vi "Read DL_param.vi"(8 "error in (no error)":errorcluster, 11 "Control-Client in":refnum<class "Control-Client.lvclass">) -> (0 "error out":errorcluster, 2 "DL_param":T1={"min I, mm"=-900.0, "max I, mm"=100.0, "Real Optical 0, ps"=480.0, "min II, mm"=-70.0, "max II, mm "=50.0}, 3 "Control-Client out":refnum<class "Control-Client.lvclass">)   [LabVIEW 2015, in "Control-Client.lvclass"]
uses:
  Control-Client.lvclass
  Control-Client.lvclass/Control-Client.ctl
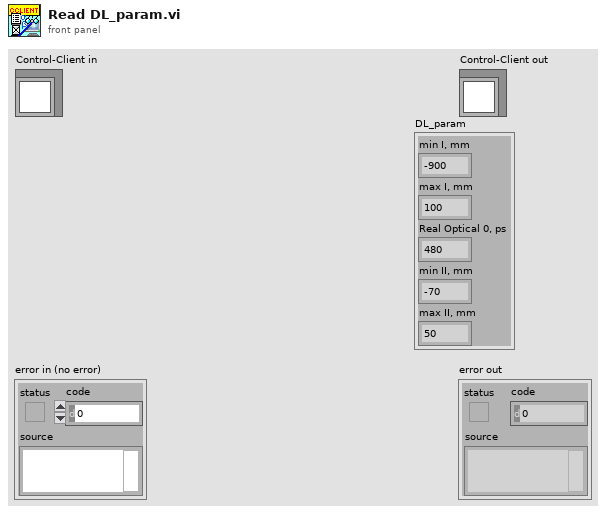
[diagram p1: front panel]
types:
  T1 = cluster{"min I, mm":dbl, "max I, mm":dbl, "Real Optical 0, ps":dbl, "min II, mm":dbl, "max II, mm ":dbl}
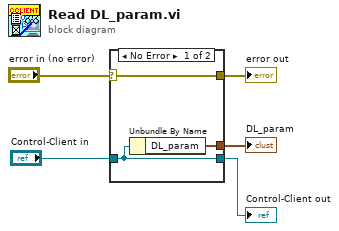
[diagram p0: block diagram]
diagram:
  n1 = case shown="No Error" "error in (no error)" {
    selector: "error in (no error)" -> [w8 w9]
    tunnel: [w8 w9] -> w4
    tunnel: [w7 w10] -> w2
    tunnel: "Control-Client in" -> [w7 w10]
    tunnel: [w6 _] -> w1
    frame No Error {
      n2 = Unbundle By Name(w7) -> ("DL_param"=w6:T1)
    }
    frame Error {
    }
  }
  "error out" <- w4
  "Control-Client out" <- w2
  "DL_param" <- w1
